vi "Obtain Notifier.vi"(8 "error in (no error)":errorcluster, 11 "CVT_Boolean in":refnum<class "CVT_Boolean.lvclass">) -> (0 "error out":errorcluster, 3 "CVT_Boolean out":refnum<class "CVT_Boolean.lvclass">)   [LabVIEW 2024, in "Current Value Table.lvlib" / "CVT_Boolean.lvclass"]
uses:
  CVT_Boolean.lvclass
  CVT_Boolean.lvclass/CVT_Boolean.ctl
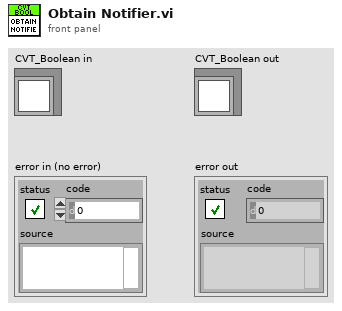
[diagram p1: front panel]
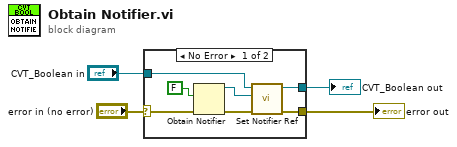
[diagram p0: block diagram]
diagram:
  n1 = case shown="No Error" "error in (no error)" {
    selector: "error in (no error)" -> [w6 w13]
    tunnel: [w8 w13] -> w3
    tunnel: [w9 w12] -> w1
    tunnel: "CVT_Boolean in" -> [w10 w12]
    frame No Error {
      n2 = Obtain Notifier(notification data type=FALSE ("element data type"), error in (no error)=w6) -> (notifier out=w11:refnum<notifier>, error out=w7:errorcluster)  [unwired: 2 in, 1 out]
      n3 = call-dynamic "Set Notifier Ref.vi"("error in (no error)"=w7, "notifier in"=w11, "CVT_Boolean in"=w10) -> ("error out"=w8:errorcluster, "CVT_Boolean out"=w9:refnum<class "CVT_Boolean.lvclass">)  [unwired: 7 in]
    }
    frame Error {
    }
  }
  "error out" <- w3
  "CVT_Boolean out" <- w1
